vi "AutoLeftDrive.vi"() -> ()   [LabVIEW 2016]
panel:
  in  "Auto Left Drive contr":dbl
  out "Auto Left Drive indic":dbl
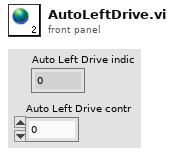
[diagram p1: front panel]
diagram:
